vi "Import Contacts.vi"(8 "error in (no error)":errorcluster, 11 "Contacts":T1[](array[typedef])) -> (0 "error out":errorcluster, 3 "Contacts out":T1[](array[typedef]))   [LabVIEW 2014, in "Map Data.lvlib"]
doc: "Imports one or more contacts into the address book data store. The output clusters will contain the ID of the new contacts."
uses:
  Map Data.lvlib
  MapCommand.ctl
  MapDatas.ctl
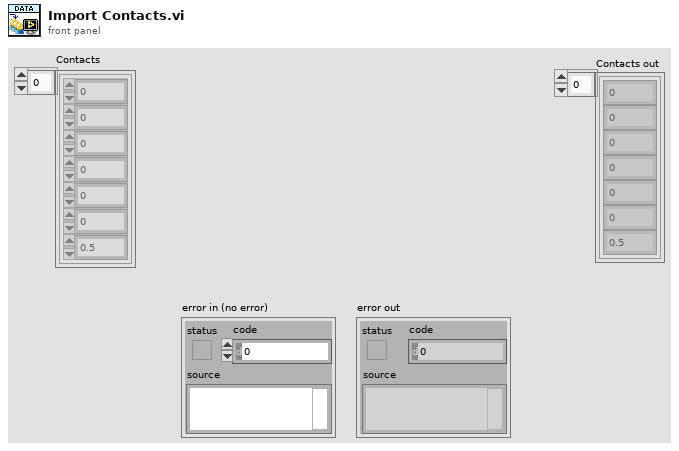
[diagram p1: front panel]
types:
  T1 = typedef "Map Data.lvlib/MapDatas.ctl" = cluster{"X":dbl, "Y":dbl, "Z":dbl, "heading":dbl, "X2":dbl, "Y2":dbl, "Z2":dbl}
  T2 = typedef "Map Data.lvlib/MapCommand.ctl" = enum16{"Load", "Update Cursor", "Save", "Get All Data", "Get Single Data", "Set Single Data", "Delete All", "Remove Single Data", "Set Favorite Status", "Is Data Modified", "Import Data"}
  T3 = typedef "Map Data.lvlib/All-Lines.ctl" = T4[]
  T4 = typedef "Map Data.lvlib/LineCluster.ctl" = cluster{"Line name":string, "Line array":cluster{"X":dbl, "Y":dbl, "Z":dbl}[], "Line connections":T5[]}
  T5 = typedef "LineConnection.ctl" = cluster{"Index":i32, "Switch Pos":cluster{"X":dbl, "Y":dbl, "Z":dbl}, "Switch operational":bool, "Switch State":bool, "Connection Index":i32, "Connection Pos":cluster{"X":dbl, "Y":dbl, "Z":dbl}, "LinePos Index":i32, "ConnectPos Index":i32, "Same direction?":bool, "Manual Overide":bool, "Manual State":bool}
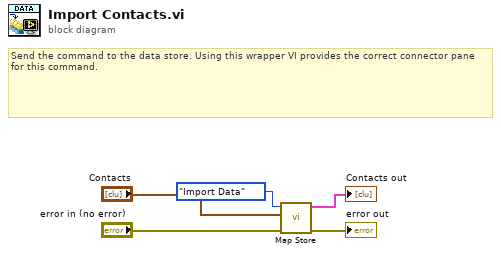
[diagram p0: block diagram]
diagram:
  # "Send the command to the data store. Using this wrapper VI provides the correct connector pane for this command."
  n1 = call "Map Store.vi"("error in (no error)"="error in (no error)", "All Lines"="Contacts", "Command"=MapCommand."Import Data") -> ("error out"=→"error out":errorcluster, "All Lines out"=→"Contacts out":T3)  [unwired: 5 in, 2 out]
